vi "TxPkt - Add Packet.vi"(8 "error in (no error)":errorcluster, 9 "New Packet ID":i32, 10 "New Packet Name":string, 11 "Item Ref in":T1=18446744073709551615 format="%.0x") -> (0 "error out":errorcluster, 2 "New Packet Ref":T1=18446744073709551615 format="%.0x", 3 "Item Ref Out":T1=18446744073709551615 format="%.0x")   [LabVIEW 2016, in "UDP-Custom-Device System Explorer.lvlib"]
uses:
  UDP-Custom-Device System Explorer.lvlib
  <vilib>/NI Veristand/Custom Device API/Custom Device Item Ref.ctl
  Shared/Constants.vi
  Shared/UDP-Custom-Device Shared.lvlib
  <vilib>/NI VeriStand/Custom Device API/Custom Device API.lvlib
  Property Accessors/Shared Section Accessors.lvlib
  Property Accessors/Shared Packet Accessors.lvlib
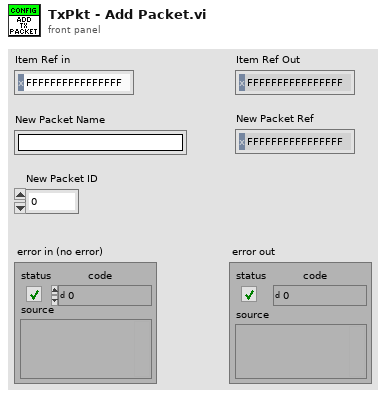
[diagram p1: front panel]
types:
  T1 = typedef "Custom Device API.lvlib/Custom Device Item Ref.ctl" = u64
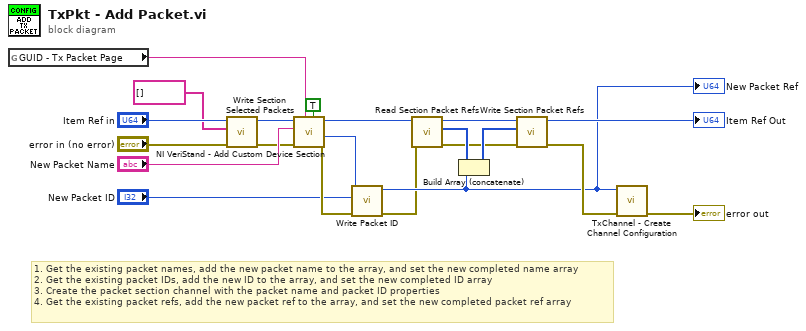
[diagram p0: block diagram]
diagram:
  # "1. Get the existing packet names, add the new packet name to the array, and set the new completed name array\n2. Get the existing packet IDs, add the new ID to the array, and set the new completed ID array\n3. Create the packet section channel with the packet name and packet ID properties\n4. Get the existing packet refs, add the new packet ref to the array, and set the new completed packet ref array"
  n1 = global read "Constants.vi" "GUID - Tx Packet Page"() -> (w20:string)
  n2 = call "Write Section Selected Packets.vi"("error in (no error)"="error in (no error)", "Selected Packets"=string[] [] ("Value"), "Node Ptr"="Item Ref in") -> ("error out"=w8:errorcluster, "Node Ptr out"=w7:T1)  [unwired: 7 in]
  n3 = call <vilib>:"NI VeriStand - Add Custom Device Section.vi"("Highlight? (F)"=TRUE, "GUID (Default Section)"=w20, "error in (no error)"=w8, "Section Name"="New Packet Name", "Parent Ref in"=w7) -> ("error out"=w3:errorcluster, "Section Ptr"=w5:T1, "Parent Ref out"=w17:T1)  [unwired: 3 in, 1 out]
  n4 = call "Write Packet ID.vi"("error in (no error)"=w3, "Packet ID"="New Packet ID", "Node Ptr"=w5) -> ("error out"=w2:errorcluster, "Node Ptr out"=w4:T1)  [unwired: 7 in]
  "New Packet Ref" <- w4
  n5 = call "Read Section Packet Refs.vi"("error in (no error)"=w2, "Node Ptr"=w17) -> ("error out"=w13:errorcluster, "Dependent Node Refs"=w15:T1[], "Node Ptr out"=w16:T1)  [unwired: 7 in]
  n6 = Build Array (concatenate)(w15, w4) -> (w14:T1[])
  n7 = call "Write Section Packet Refs.vi"("error in (no error)"=w13, "Dependent Node Refs"=w14, "Node Ptr"=w16) -> ("error out"=w11:errorcluster, "Node Ptr out"=→"Item Ref Out":T1)  [unwired: 7 in]
  n8 = call "TxChannel - Create Channel Configuration.vi"("error in (no error)"=w11, "Parent Packet Ref"=w4) -> ("error out"=→"error out":errorcluster)  [unwired: 8 in, 1 out]
